vi "XMLCreate.vi"(8 "Error In":errorcluster, 11 "DOM document in":refnum<k20>) -> (0 "Error Out":errorcluster, 1 "server endpoint URL":string, 2 "OPC UA server refnum out":refnum<k21>, 3 "DOM document out":refnum<k20>)   [LabVIEW 2014, in "OPCUA XML.lvlib"]
uses:
  OPCUA XML.lvlib
  <vilib>/xml/Close Reference(Node).vi
  <vilib>/xml/Close Reference(NdList).vi
  <resource>/objmgr/DOMUserDefRef.rc
  <vilib>/xml/NI_XML.lvlib
  <vilib>/OPCUA/NI OPC UA Server.lvlib
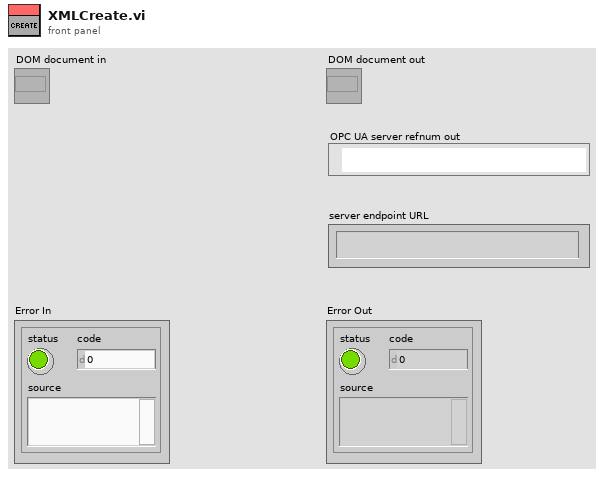
[diagram p1: front panel]
types:
  T1 = typedef "supported security policies.ctl" = cluster{"None":bool, "Sign with Basic128Rsa125":bool, "Sign and Encrypt with Basic128Rsa125":bool, "Sign with Basic256":bool, "Sign and Encrypt with Basic256":bool}
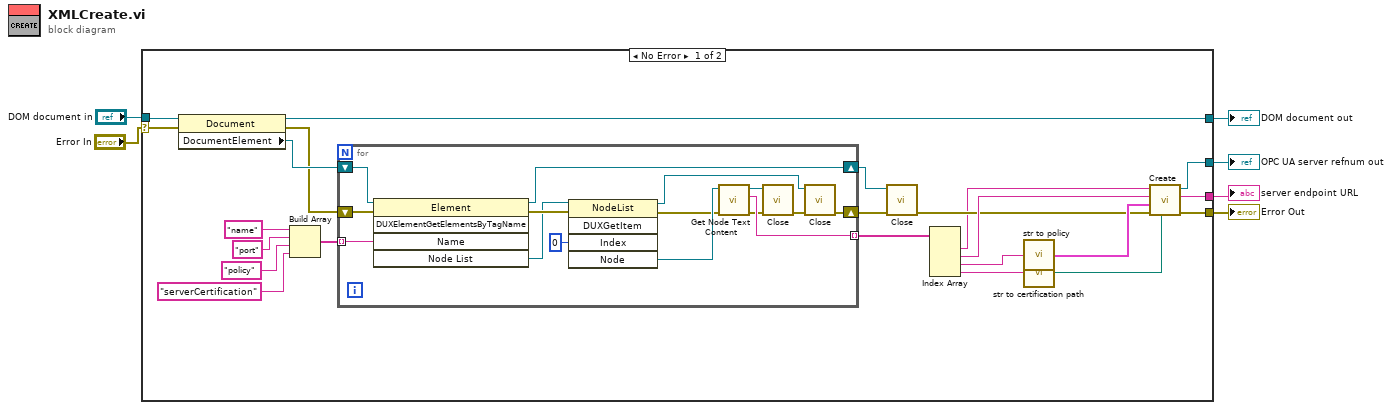
[diagram p0: block diagram]
diagram:
  n1 = case shown="No Error" "Error In" {
    selector: "Error In" -> [w29 w46]
    tunnel: [w13 w46] -> w6
    tunnel: "DOM document in" -> [w28 w45]
    tunnel: [w27 w45] -> w3
    tunnel: [w15 _] -> w1
    tunnel: [w14 _] -> w2
    frame No Error {
      n2 = property class="Document"(reference=w28, error in=w29) -> (reference out=w27:refnum<k20>, error out=w25:errorcluster, "DocumentElement"=w26:refnum<k20>)
      n3 = Build Array("name" ("Name"), "port" ("Name"), "policy" ("Name"), "serverCertification" ("Name")) -> (w20:string[])
      n4 = for {
        tunnel: w20 -> [w42] mode=indexing
        tunnel: [w37] -> w19 mode=indexing
        shift-right: [w32] -> w12
        shift-left: w25 -> [w43]
        shift-right: [w31] -> w11
        shift-left: w26 -> [w44]
        n5 = invoke class="Element" method="DUXElementGetElementsByTagName"(reference=w44, error in=w43, "Name"=w42) -> (reference out=w31:refnum<k20>, error out=w40:errorcluster, "Node List"=w39:refnum<k20>)  [unwired: 2 in, 2 out]
        n6 = invoke class="NodeList" method="DUXGetItem"(reference=w39, error in=w40, "Index"=0) -> (reference out=w33:refnum<k20>, error out=w30:errorcluster, "Node"=w38:refnum<k20>)  [unwired: 2 in, 2 out]
        n7 = call <vilib>:"Get Node Text Content.vi"("error in (no error)"=w30, "node in"=w38) -> ("error out"=w36:errorcluster, "node text"=w37:string, "node out"=w35:refnum<k20>)  [unwired: 7 out]
        n8 = call-poly <vilib>:"Close.vi"("error in (no error)"=w36, "node"=w35) -> ("error out"=w34:errorcluster)  [unwired: 7 out]
        n9 = call-poly <vilib>:"Close.vi"("error in (no error)"=w34, "node list"=w33) -> ("error out"=w32:errorcluster)  [unwired: 7 out]
      }
      n10 = call-poly <vilib>:"Close.vi"("error in (no error)"=w12, "node"=w11) -> ("error out"=w10:errorcluster)  [unwired: 7 out]
      n11 = Index Array(array=w19) -> (element #1=w9:string, element #2=w18:string, element #3=w17:string, element #4=w7:string)  [unwired: 4 in]
      n12 = call "str to policy.vi"("String"=w17) -> ("supported security policies (None)"=w16:T1)  [unwired: 6 in]
      n13 = call "str to certification path.vi"("node text"=w7) -> ("File Path Control"=w8:path)  [unwired: 4 in]
      n14 = call <vilib>:"Create.vi"("server certificate file"=w8, "error in (no error)"=w10, "supported security policies (None)"=w16, "TCP port (49580)"=w18, "OPC UA server name"=w9) -> ("error out"=w13:errorcluster, "server endpoint URL"=w14:string, "OPC UA server refnum out"=w15:refnum<k21>)  [unwired: 4 in]
    }
    frame Error {
    }
  }
  "Error Out" <- w6
  "DOM document out" <- w3
  "OPC UA server refnum out" <- w1
  "server endpoint URL" <- w2
